vi "Build Graphs.vi"(6 "High":bool, 7 "Integrator Action":dbl, 8 "PV":dbl, 9 "Setpoint":dbl, 10 "Plot 2 in":cluster{dbl[], dbl[]}, 11 "Plot 1 in":cluster{dbl[], dbl[]}) -> (2 "Plot 2 out":cluster{dbl[], dbl[]}, 3 "Plot 1 out":cluster{dbl[], dbl[]})   [LabVIEW 2015]
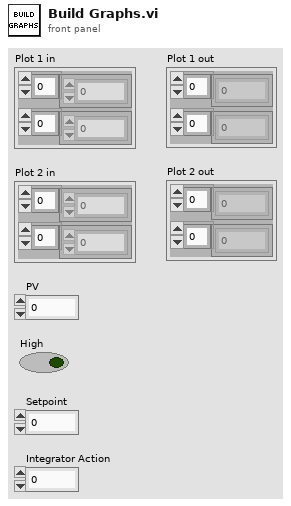
[diagram p1: front panel]
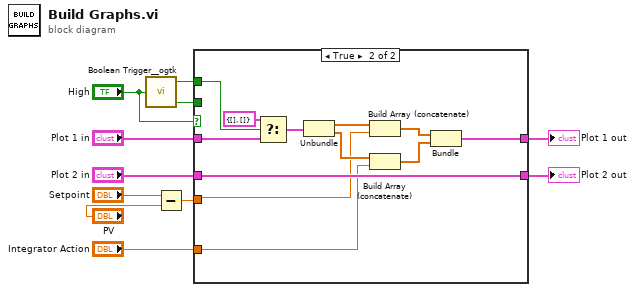
[diagram p0: block diagram]
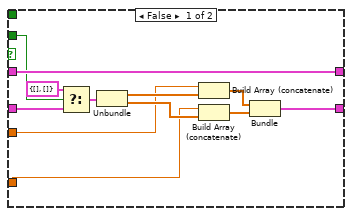
[diagram p2: hidden frame]
diagram:
  n1 = call <userlib>:"Boolean Trigger__ogtk.vi"("Boolean Input"="High") -> ("Rising Edge"=w6:bool, "Falling Edge"=w7:bool)  [unwired: 1 in]
  n2 = Subtract(x="Setpoint", y="PV") -> (x-y=w3:dbl)
  n3 = case shown="True" "High" {
    tunnel: "Plot 1 in" -> [w18 w27]
    tunnel: w3 -> [w12 w25]
    tunnel: [w18 w26] -> w8
    tunnel: "Integrator Action" -> [w13 w24]
    tunnel: "Plot 2 in" -> [w15 w28]
    tunnel: [w19 w28] -> w9
    tunnel: w6 -> [_ w29]
    tunnel: w7 -> [w17 _]
    frame False {
      n4 = Select(t=cluster{dbl[], dbl[]} {[], []}, s=w17, f=w15) -> (s? t:f=w14:cluster{dbl[], dbl[]})
      n5 = Unbundle(w14) -> (w23:dbl[], w22:dbl[])
      n6 = Build Array (concatenate)(w12, w23) -> (w21:dbl[])
      n7 = Build Array (concatenate)(w13, w22) -> (w20:dbl[])
      n8 = Bundle(w21, w20) -> (w19:cluster{dbl[], dbl[]})  [unwired: 1 in]
    }
    frame True {
      n9 = Select(t=cluster{dbl[], dbl[]} {[], []}, s=w29, f=w27) -> (s? t:f=w30:cluster{dbl[], dbl[]})
      n10 = Unbundle(w30) -> (w35:dbl[], w34:dbl[])
      n11 = Build Array (concatenate)(w35, w25) -> (w33:dbl[])
      n12 = Build Array (concatenate)(w34, w24) -> (w32:dbl[])
      n13 = Bundle(w33, w32) -> (w26:cluster{dbl[], dbl[]})  [unwired: 1 in]
    }
  }
  "Plot 2 out" <- w9
  "Plot 1 out" <- w8
